vi "Status Channel Summary Enable.vi"(0 "VISA resource name":refnum<visa-resource-name>, 7 "Channel Sum Reg (CH1-8 F:0)":T1, 11 "error in (no error)":errorcluster) -> (4 "VISA resource name out":refnum<visa-resource-name>, 15 "error out":errorcluster)   [LabVIEW 2015, in "Chroma ATE 6310.lvlib"]
doc: "Mask for selecting which bits in the Channel Event register are allowed to be summed into the CSUM bit of the Status Byte register."
uses:
  <instrlib>/Chroma ATE 6310/Chroma ATE 6310.lvlib
panel:
  # "Channel :       1          2          3          4           5          6          7          8"
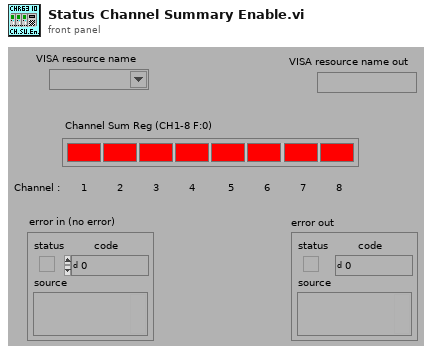
[diagram p1: front panel]
types:
  T1 = cluster{"CH1 (F:0)":bool, "CH2 (F:0)":bool, "CH3 (F:0)":bool, "CH4 (F:0)":bool, "CH5 (F:0)":bool, "CH6 (F:0)":bool, "CH7 (F:0)":bool, "CH8 (F:0)":bool}
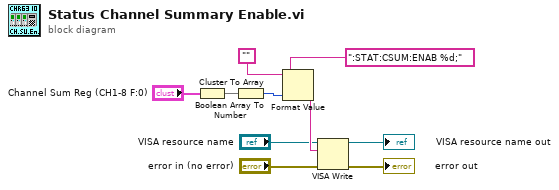
[diagram p0: block diagram]
diagram:
  n1 = Cluster To Array(cluster="Channel Sum Reg (CH1-8 F:0)") -> (array=w7:bool[])
  n2 = Boolean Array To Number(Boolean array=w7) -> (number=w6:u32)
  n3 = Format Value(string ("")="", format string=":STAT:CSUM:ENAB %d;", value (0)=w6) -> (output string=w9:string)
  n4 = VISA Write(VISA resource name="VISA resource name", write buffer=w9, error in (no error)="error in (no error)") -> (VISA resource name out=→"VISA resource name out":refnum<visa-resource-name>, error out=→"error out":errorcluster)  [unwired: 1 out]
